vi "MV3D RGBD Open U3Device.vi"(10 "pstU3DeviceInfo":T1, 11 "handle":u32) -> (1 "function return":i32, 2 "pstU3DeviceInfo out":T1, 3 "handle out":u32)   [LabVIEW 2015, in "Mv3dRgbdEx.lvlib"]
doc: "MV3D_RGBD_API_Ex MV3D_RGBD_STATUS MV3D_RGBD_OpenU3Device(HANDLE *handle, MV3D_RGBD_U3DEVICE_INFO* pstU3DeviceInfo = NULL);"
uses:
  <userlib>/Mv3dRgbdEx/Mv3dRgbdEx.lvlib
  <userlib>/Mv3dRgbdEx/Mv3dRgbdEx.dll
types:
  T1 = cluster{"chManufacturerName[0]":i8, "chManufacturerName[1]":i8, "chManufacturerName[2]":i8, "chManufacturerName[3]":i8, "chManufacturerName[4]":i8, "chManufacturerName[5]":i8, "chManufacturerName[6]":i8, "chManufacturerName[7]":i8, "chManufacturerName[8]":i8, "chManufacturerName[9]":i8, "chManufacturerName[10]":i8, "chManufacturerName[11]":i8, "chManufacturerName[12]":i8, "chManufacturerName[13]":i8, "chManufacturerName[14]":i8, "chManufacturerName[15]":i8, "chManufacturerName[16]":i8, "chManufacturerName[17]":i8, "chManufacturerName[18]":i8, "chManufacturerName[19]":i8, "chManufacturerName[20]":i8, "chManufacturerName[21]":i8, "chManufacturerName[22]":i8, "chManufacturerName[23]":i8, "chManufacturerName[24]":i8, "chManufacturerName[25]":i8, "chManufacturerName[26]":i8, "chManufacturerName[27]":i8, "chManufacturerName[28]":i8, "chManufacturerName[29]":i8, "chManufacturerName[30]":i8, "chManufacturerName[31]":i8, "chModelName[0]":i8, "chModelName[1]":i8, "chModelName[2]":i8, "chModelName[3]":i8, "chModelName[4]":i8, "chModelName[5]":i8, "chModelName[6]":i8, "chModelName[7]":i8, "chModelName[8]":i8, "chModelName[9]":i8, "chModelName[10]":i8, "chModelName[11]":i8, "chModelName[12]":i8, "chModelName[13]":i8, "chModelName[14]":i8, "chModelName[15]":i8, "chModelName[16]":i8, "chModelName[17]":i8, "chModelName[18]":i8, "chModelName[19]":i8, "chModelName[20]":i8, "chModelName[21]":i8, "chModelName[22]":i8, "chModelName[23]":i8, "chModelName[24]":i8, "chModelName[25]":i8, "chModelName[26]":i8, "chModelName[27]":i8, "chModelName[28]":i8, "chModelName[29]":i8, "chModelName[30]":i8, "chModelName[31]":i8, "chDeviceVersion[0]":i8, "chDeviceVersion[1]":i8, "chDeviceVersion[2]":i8, "chDeviceVersion[3]":i8, "chDeviceVersion[4]":i8, "chDeviceVersion[5]":i8, "chDeviceVersion[6]":i8, "chDeviceVersion[7]":i8, "chDeviceVersion[8]":i8, "chDeviceVersion[9]":i8, "chDeviceVersion[10]":i8, "chDeviceVersion[11]":i8, "chDeviceVersion[12]":i8, "chDeviceVersion[13]":i8, "chDeviceVersion[14]":i8, "chDeviceVersion[15]":i8, "chDeviceVersion[16]":i8, "chDeviceVersion[17]":i8, "chDeviceVersion[18]":i8, "chDeviceVersion[19]":i8, "chDeviceVersion[20]":i8, "chDeviceVersion[21]":i8, "chDeviceVersion[22]":i8, "chDeviceVersion[23]":i8, "chDeviceVersion[24]":i8, "chDeviceVersion[25]":i8, "chDeviceVersion[26]":i8, "chDeviceVersion[27]":i8, "chDeviceVersion[28]":i8, "chDeviceVersion[29]":i8, "chDeviceVersion[30]":i8, "chDeviceVersion[31]":i8, "chManufacturerSpecificInfo[0]":i8, "chManufacturerSpecificInfo[1]":i8, "chManufacturerSpecificInfo[2]":i8, "chManufacturerSpecificInfo[3]":i8, "chManufacturerSpecificInfo[4]":i8, "chManufacturerSpecificInfo[5]":i8, "chManufacturerSpecificInfo[6]":i8, "chManufacturerSpecificInfo[7]":i8, "chManufacturerSpecificInfo[8]":i8, "chManufacturerSpecificInfo[9]":i8, "chManufacturerSpecificInfo[10]":i8, "chManufacturerSpecificInfo[11]":i8, "chManufacturerSpecificInfo[12]":i8, "chManufacturerSpecificInfo[13]":i8, "chManufacturerSpecificInfo[14]":i8, "chManufacturerSpecificInfo[15]":i8, "chManufacturerSpecificInfo[16]":i8, "chManufacturerSpecificInfo[17]":i8, "chManufacturerSpecificInfo[18]":i8, "chManufacturerSpecificInfo[19]":i8, "chManufacturerSpecificInfo[20]":i8, "chManufacturerSpecificInfo[21]":i8, "chManufacturerSpecificInfo[22]":i8, "chManufacturerSpecificInfo[23]":i8, "chManufacturerSpecificInfo[24]":i8, "chManufacturerSpecificInfo[25]":i8, "chManufacturerSpecificInfo[26]":i8, "chManufacturerSpecificInfo[27]":i8, "chManufacturerSpecificInfo[28]":i8, "chManufacturerSpecificInfo[29]":i8, "chManufacturerSpecificInfo[30]":i8, "chManufacturerSpecificInfo[31]":i8, "chManufacturerSpecificInfo[32]":i8, "chManufacturerSpecificInfo[33]":i8, "chManufacturerSpecificInfo[34]":i8, "chManufacturerSpecificInfo[35]":i8, "chManufacturerSpecificInfo[36]":i8, "chManufacturerSpecificInfo[37]":i8, "chManufacturerSpecificInfo[38]":i8, "chManufacturerSpecificInfo[39]":i8, "chManufacturerSpecificInfo[40]":i8, "chManufacturerSpecificInfo[41]":i8, "chManufacturerSpecificInfo[42]":i8, "chManufacturerSpecificInfo[43]":i8, "chManufacturerSpecificInfo[44]":i8, "chManufacturerSpecificInfo[45]":i8, "chManufacturerSpecificInfo[46]":i8, "chManufacturerSpecificInfo[47]":i8, "chSerialNumber[0]":i8, "chSerialNumber[1]":i8, "chSerialNumber[2]":i8, "chSerialNumber[3]":i8, "chSerialNumber[4]":i8, "chSerialNumber[5]":i8, "chSerialNumber[6]":i8, "chSerialNumber[7]":i8, "chSerialNumber[8]":i8, "chSerialNumber[9]":i8, "chSerialNumber[10]":i8, "chSerialNumber[11]":i8, "chSerialNumber[12]":i8, "chSerialNumber[13]":i8, "chSerialNumber[14]":i8, "chSerialNumber[15]":i8, "chUserDefinedName[0]":i8, "chUserDefinedName[1]":i8, "chUserDefinedName[2]":i8, "chUserDefinedName[3]":i8, "chUserDefinedName[4]":i8, "chUserDefinedName[5]":i8, "chUserDefinedName[6]":i8, "chUserDefinedName[7]":i8, "chUserDefinedName[8]":i8, "chUserDefinedName[9]":i8, "chUserDefinedName[10]":i8, "chUserDefinedName[11]":i8, "chUserDefinedName[12]":i8, "chUserDefinedName[13]":i8, "chUserDefinedName[14]":i8, "chUserDefinedName[15]":i8, "enDeviceType":i32, "nVendorId":u32, "nProductId":u32, "enUsbProtocol":i32, "chDeviceGUID[0]":i8, "chDeviceGUID[1]":i8, "chDeviceGUID[2]":i8, "chDeviceGUID[3]":i8, "chDeviceGUID[4]":i8, "chDeviceGUID[5]":i8, "chDeviceGUID[6]":i8, "chDeviceGUID[7]":i8, "chDeviceGUID[8]":i8, "chDeviceGUID[9]":i8, "chDeviceGUID[10]":i8, "chDeviceGUID[11]":i8, "chDeviceGUID[12]":i8, "chDeviceGUID[13]":i8, "chDeviceGUID[14]":i8, "chDeviceGUID[15]":i8, "chDeviceGUID[16]":i8, "chDeviceGUID[17]":i8, "chDeviceGUID[18]":i8, "chDeviceGUID[19]":i8, "chDeviceGUID[20]":i8, "chDeviceGUID[21]":i8, "chDeviceGUID[22]":i8, "chDeviceGUID[23]":i8, "chDeviceGUID[24]":i8, "chDeviceGUID[25]":i8, "chDeviceGUID[26]":i8, "chDeviceGUID[27]":i8, "chDeviceGUID[28]":i8, "chDeviceGUID[29]":i8, "chDeviceGUID[30]":i8, "chDeviceGUID[31]":i8, "chDeviceGUID[32]":i8, "chDeviceGUID[33]":i8, "chDeviceGUID[34]":i8, "chDeviceGUID[35]":i8, "chDeviceGUID[36]":i8, "chDeviceGUID[37]":i8, "chDeviceGUID[38]":i8, "chDeviceGUID[39]":i8, "chDeviceGUID[40]":i8, "chDeviceGUID[41]":i8, "chDeviceGUID[42]":i8, "chDeviceGUID[43]":i8, "chDeviceGUID[44]":i8, "chDeviceGUID[45]":i8, "chDeviceGUID[46]":i8, "chDeviceGUID[47]":i8, "chDeviceGUID[48]":i8, "chDeviceGUID[49]":i8, "chDeviceGUID[50]":i8, "chDeviceGUID[51]":i8, "chDeviceGUID[52]":i8, "chDeviceGUID[53]":i8, "chDeviceGUID[54]":i8, "chDeviceGUID[55]":i8, "chDeviceGUID[56]":i8, "chDeviceGUID[57]":i8, "chDeviceGUID[58]":i8, "chDeviceGUID[59]":i8, "chDeviceGUID[60]":i8, "chDeviceGUID[61]":i8, "chDeviceGUID[62]":i8, "chDeviceGUID[63]":i8, "nReserved[0]":u8, "nReserved[1]":u8, "nReserved[2]":u8, "nReserved[3]":u8, "nReserved[4]":u8, "nReserved[5]":u8, "nReserved[6]":u8, "nReserved[7]":u8, "nReserved[8]":u8, "nReserved[9]":u8, "nReserved[10]":u8, "nReserved[11]":u8, "nReserved[12]":u8, "nReserved[13]":u8, "nReserved[14]":u8, "nReserved[15]":u8}
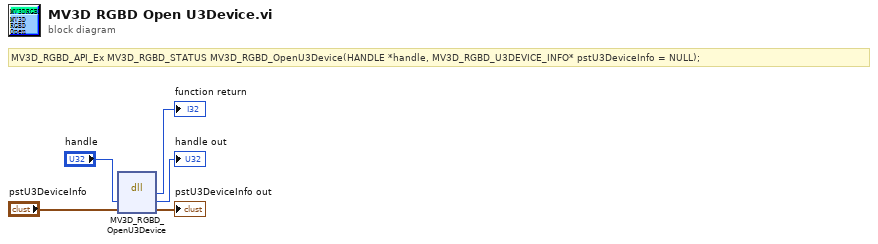
[diagram p0: block diagram]
diagram:
  # "MV3D_RGBD_API_Ex MV3D_RGBD_STATUS MV3D_RGBD_OpenU3Device(HANDLE *handle, MV3D_RGBD_U3DEVICE_INFO* pstU3DeviceInfo = NULL);"
  n1 = dll-call lib="C:/Program Files (x86)/National Instruments/LabVIEW 2015/user.lib/Mv3dRgbdEx/Mv3dRgbdEx.*" fn="MV3D_RGBD_OpenU3Device"("handle"="handle", "pstU3DeviceInfo"="pstU3DeviceInfo") -> (→"function return":i32, "handle"=→"handle out":u32, "pstU3DeviceInfo"=→"pstU3DeviceInfo out":T1)  [unwired: 3 in, 2 out]
